vi "Close.vi"(8 "error in":errorcluster, 11 "Synnax Client in":refnum<class "Synnax Client.lvclass">) -> (0 "error out":errorcluster)   [LabVIEW 2026, in "synnax_clib.lvlib" / "Synnax Client.lvclass"]
uses:
  Synnax Client.lvclass
  Synnax Client.lvclass/Synnax Client.ctl
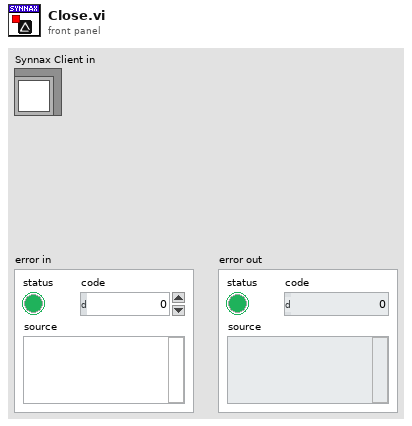
[diagram p1: front panel]
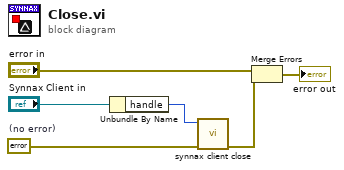
[diagram p0: block diagram]
diagram:
  w1 = errorcluster {"status"=FALSE, "code"=0, "source"=""}  # (no error)
  n1 = Unbundle By Name("Synnax Client in") -> ("handle"=w2:u64)
  n2 = call "synnax client close.vi"("error in"=w1, "client"=w2) -> ("error out"=w6:errorcluster)  [unwired: 9 in]
  n3 = Merge Errors("error in", w6) -> (→"error out":errorcluster)
